vi "Joystick_test.vi"() -> ()   [LabVIEW 2017]
uses:
  NationalInstruments.VeriStand.SystemStorage
  NationalInstruments.VeriStand.SystemStorageUI
  <vilib>/Utility/file.llb/Read Delimited Spreadsheet (string).vi
  <vilib>/Utility/inputDevices.llb/joystickAcquire.vi
  <vilib>/NI Veristand/Execution/Workspace/NI VeriStand - Set Multiple Channel Values.vi
  <vilib>/NI Veristand/Execution/Workspace/NI_VS Workspace ExecutionAPI.lvlib
  <vilib>/NI Veristand/UI Controls/Single Node Browser/NI_VS UI Single Node Browser.lvlib
panel:
  in  "Single Node Browser":refnum<k24>
  out "FChannel":string[](array[string])
  out "Joystick Values":i32[](array[numeric])
  out "error out":errorcluster
  in  "Random?":bool=TRUE
  in  "Stop":bool
  in  "NIVS.System Definition Root":refnum<k24>
  in  "NIVS.Project File Path":path
  in  "NIVS.Workspace Event":refnum<event-registration>
  in  "NIVS.Gateway IP Address":string
  in  "NIVS.INI File Path":path
  # "Use this example as a template to create custom tools for the NI VeriStand Workspace. This example shows the use of the NI VeriStand API and UI controls to set and get data.\n\nRun this example by adding this VI as a Workspace Tool item. For Help adding Workspace Tool items, please reference the NI VeriStand Help."
  # "This is the file path to the VeriStand system definition file. You can read or write to the file using the System Definition API."
  # "This is the root reference to the active System Definition file. You could use this to read the configuration or populate a tree with channels. You are free to close this reference, but it will be closed for you if you don't."
  # "This is the IP Address of the VeriStand Gateway to which the Workspace is connected. Use this to open all the .NET Manager references. Usually the Gateway is running on localhost, but it could be running on a neighbor's machine."
  # "This registered string User Event is used to help instruct your tool to shut down when the Workspace is closing."
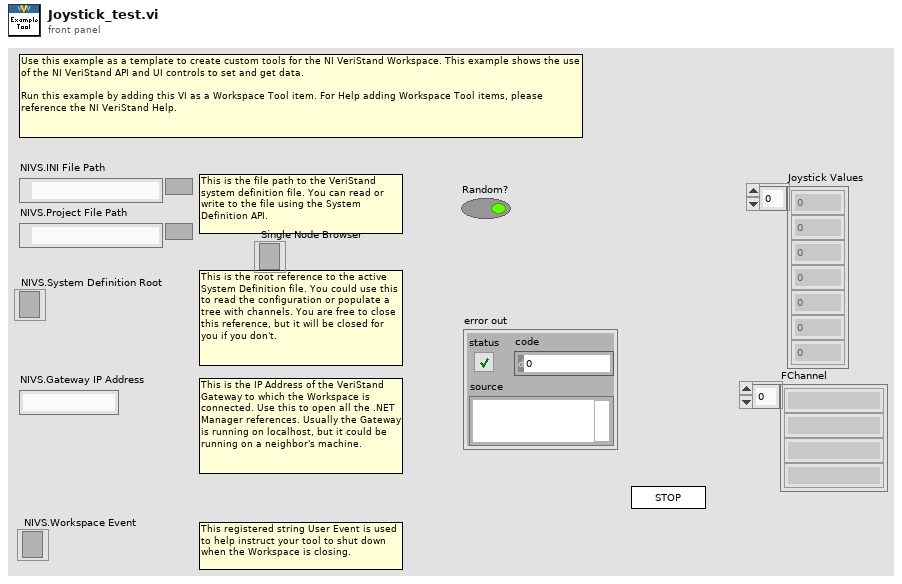
[diagram p1: front panel]
types:
  T1 = typedef "NI_VS UI Single Node Browser.lvlib/Callback Type.ctl" = cluster{"Net Callbacks":refnum<k27>[], "Event":refnum<user-event>}
  T2 = typedef "NI_VS Workspace ExecutionAPI.lvlib/WorkspaceAPI.ctl" = refnum<k24>
  T3 = typedef "NI_VS Workspace ExecutionAPI.lvlib/SystemStateEventRef.ctl" = cluster{"CustDatRef":refnum<user-event>, "EvtRef":refnum<k27>, "Target State User Event":refnum<user-event>}
  T4 = typedef "NI_VS Workspace ExecutionAPI.lvlib/SystemStateRegEventRef.ctl" = refnum<event-registration>
  T5 = cluster{"NIVS.Workspace Event":refnum<event-registration>, "Event Registration Refnum":refnum<event-registration>, "SystemChangeEventRef":T4}
  T6 = cluster{"X axis":i32, "Y axis":i32, "Z axis":i32, "X axis rotation":i32, "Y axis rotation":i32, "Z axis rotation":i32, "U axis":i32, "V axis":i32}
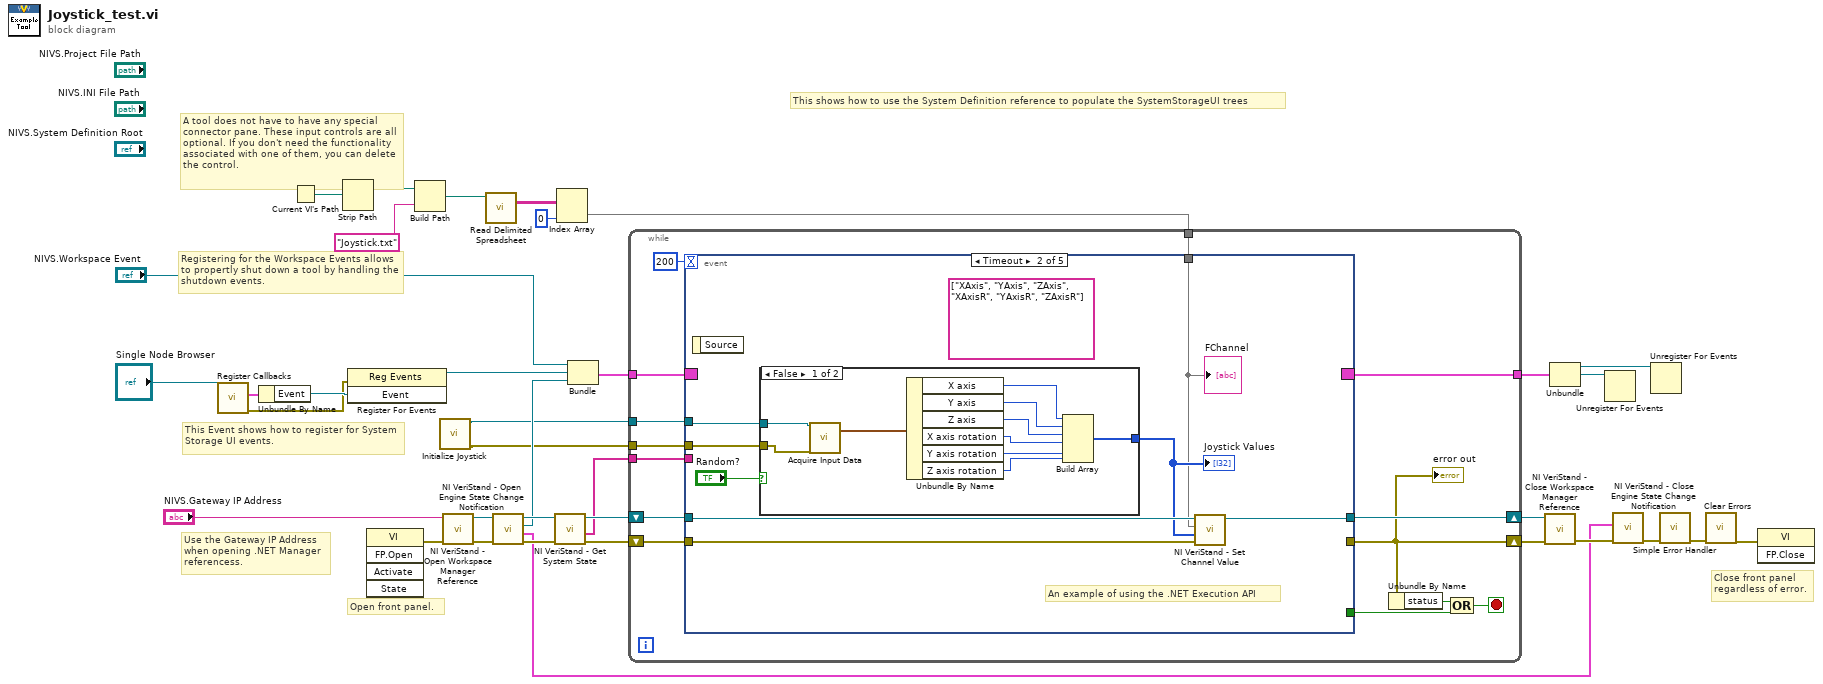
[diagram p0: block diagram]
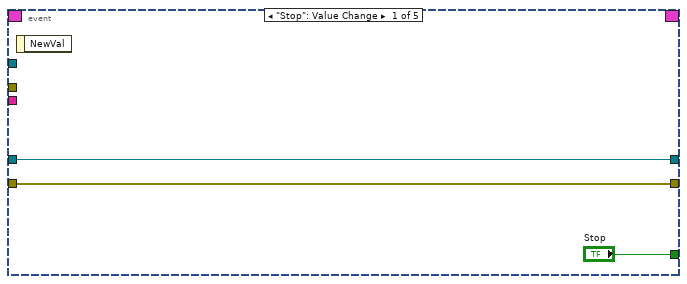
[diagram p2: hidden frame]
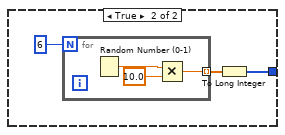
[diagram p3: hidden frame]
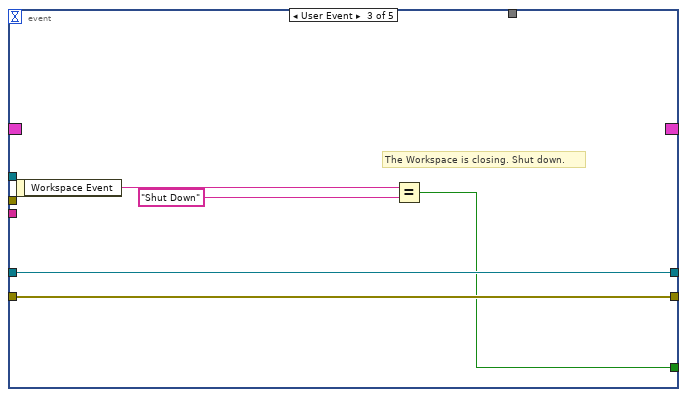
[diagram p4: hidden frame]
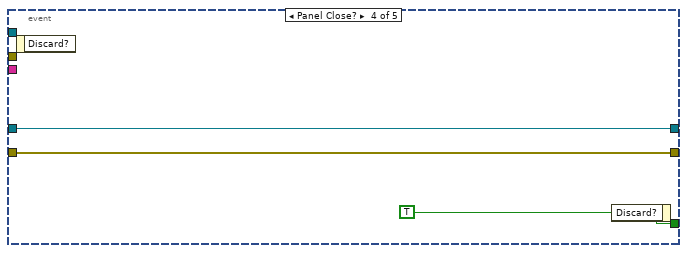
[diagram p5: hidden frame]
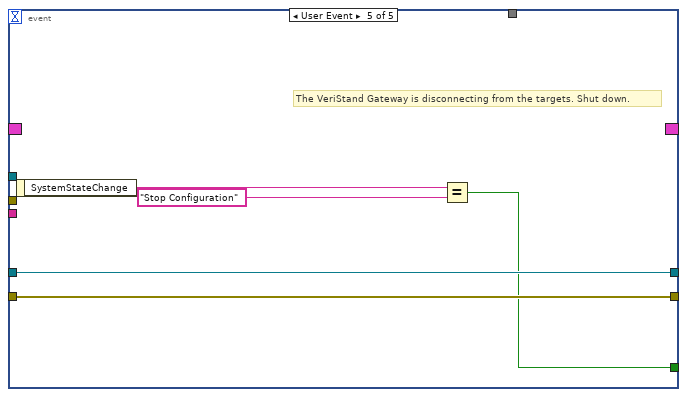
[diagram p6: hidden frame]
diagram:
  # "This Event shows how to register for System Storage UI events."
  # "Use the Gateway IP Address when opening .NET Manager referencess."
  # "A tool does not have to have any special connector pane. These input controls are all optional. If you don't need the functionality associated with one of them, you can delete the control."
  # "This shows how to use the System Definition reference to populate the SystemStorageUI trees"
  # "Registering for the Workspace Events allows to propertly shut down a tool by handling the shutdown events."
  # "Close front panel\nregardless of error."
  # "Open front panel."
  n1 = call <vilib>:"Register Callbacks.vi"("Single Node Browser"="Single Node Browser") -> ("error out"=w1:errorcluster, "Callbacks"=w12:T1)  [unwired: 8 in, 1 out]
  n2 = Unbundle By Name(w12) -> ("Event"=w11:refnum<user-event>)
  n3 = Current VI's Path() -> (path=w10:path)
  n4 = Strip Path(path=w10) -> (stripped path=w9:path)  [unwired: 1 out]
  n5 = register-events(error in=w1, w11) -> (reference out=w15:refnum<event-registration>)  [unwired: 1 in, 1 out]
  n6 = invoke class="VI" method="FP.Open"() -> (error out=w19:errorcluster)  [unwired: 5 in, 4 out]
  n7 = Build Path(base path=w9, name or relative path="Joystick.txt") -> (appended path=w7:path)
  n8 = call <vilib>:"Initialize Joystick.vi"() -> ("error out"=w2:errorcluster, "device ID"=w3:refnum<k1>)  [unwired: 10 in]
  n9 = call <vilib>:"NI VeriStand - Open Workspace Manager Reference.vi"("error in (no error)"=w19, "Gateway IP Address (\"\": localhost)"="NIVS.Gateway IP Address") -> ("error out"=w30:errorcluster, "WorkspaceManager"=w31:T2)  [unwired: 8 in]
  n10 = call-poly <vilib>:"Read Delimited Spreadsheet.vi"("file path (dialog if empty)"=w7) -> ("all rows"=w6:string[][])  [unwired: 9 in, 5 out]
  n11 = call <vilib>:"NI VeriStand - Open Engine State Change Notification.vi"("error in (no error)"=w30, "WorkspaceManager in"=w31) -> ("error out"=w35:errorcluster, "SystemStateRefs"=w24:T3, "SystemChangeEventRef"=w14:T4, "WorkspaceManager out"=w36:T2)  [unwired: 6 in]
  n12 = call <vilib>:"NI VeriStand - Get System State.vi"("error in (no error)"=w35, "WorkspaceManager in"=w36) -> ("error out"=w22:errorcluster, "Targets"=w21:string[], "WorkspaceManager  out"=w23:T2)  [unwired: 5 in, 2 out]
  n13 = Index Array(array=w6, index (col)=0 ("disabled index (col)")) -> (element=w4:string[])  [unwired: 1 in]
  n14 = Bundle("NIVS.Workspace Event"="NIVS.Workspace Event", "Event Registration Refnum"=w15, "SystemChangeEventRef"=w14) -> (w29:T5)  [unwired: 1 in]
  n15 = while {
    tunnel: w29 -> [w50]
    tunnel: [w49] -> w28
    shift-right: [w42] -> w32
    shift-left: w22 -> [w47]
    shift-right: [w46] -> w33
    shift-left: w23 -> [w48]
    tunnel: w21 -> [w44]
    tunnel: w2 -> [w39]
    tunnel: w3 -> [w38]
    tunnel: w4 -> [w37]
    stop <- w40 stop-if-true
    n16 = event shown="[1] Timeout" {
      selector: w50 -> [_ _ _ _ _]
      dyn-events: [_ _ _ _ _] -> w49
      timeout: 200 -> [_ _ _ _ _]
      tunnel: ["Stop" _ w78 w83 w86] -> w41
      tunnel: w48 -> [w52 w61 w81 w84 w89]
      tunnel: w47 -> [w53 w60 w82 w85 w90]
      tunnel: [w53 _ w82 w85 w90] -> w42
      tunnel: [w52 w59 w81 w84 w89] -> w46
      tunnel: w44 -> [_ _ _ _ _]
      tunnel: w39 -> [_ w56 _ _ _]
      tunnel: w38 -> [_ w58 _ _ _]
      tunnel: w37 -> [_ w54 _ _ _]
      event "Stop": Value Change {
        n17 = event-data() -> ()  [unwired: 1 in, 1 out]
      }
      event Timeout {
        (unwired) string[] ["XAxis", "YAxis", "ZAxis", "XAxisR", "YAxisR", "ZAxisR"] ("Channels")
        # "An example of using the .NET Execution API"
        n18 = event-data() -> ()  [unwired: 1 in, 1 out]
        n19 = case shown="False" "Random?" {
          tunnel: [w65 w72] -> w57
          tunnel: w58 -> [w64 _]
          tunnel: w56 -> [w63 _]
          frame False {
            n20 = call-poly <vilib>:"Acquire Input Data.vi"("device ID"=w64, "error in (no error)"=w63) -> ("axis info"=w62:T6)  [unwired: 13 in, 4 out]
            n21 = Unbundle By Name(w62) -> ("X axis"=w71:i32, "Y axis"=w70:i32, "Z axis"=w69:i32, "X axis rotation"=w68:i32, "Y axis rotation"=w67:i32, "Z axis rotation"=w66:i32)
            n22 = Build Array(w71, w70, w69, w68, w67, w66) -> (w65:i32[])
          }
          frame True {
            n23 = for {
              N: 6 -> [_]
              tunnel: [w76] -> w74 mode=indexing
              n24 = Random Number (0-1)() -> (number: 0 to 1=w77:dbl)
              n25 = Multiply(x=w77, y=10.0) -> (x*y=w76:dbl)
            }
            n26 = To Long Integer(number=w74) -> (32bit integer=w72:i32[])
          }
        }
        "Joystick Values" <- w57
        n27 = call-poly <vilib>:"NI VeriStand - Set Channel Value.vi"("error in (no error)"=w60, "Values"=w57, "Channels"=w54, "WorkspaceManager in"=w61) -> ("WorkspaceManager out"=w59:T2)  [unwired: 6 in, 1 out]
        "FChannel" <- w54
      }
      event User Event {
        # "The Workspace is closing. Shut down."
        n28 = event-data() -> ("Workspace Event"=w80:string)  [unwired: 1 in]
        n29 = Equal?(x=w80, y="Shut Down") -> (x = y?=w78:bool)
      }
      event Panel Close? {
        w83 = TRUE ("Discard?")
        n30 = event-data() -> ()  [unwired: 1 in, 1 out]
        n31 = event-data("Discard?"=w83) -> ()  [unwired: 1 in, 1 out]
      }
      event User Event {
        # "The VeriStand Gateway is disconnecting from the targets. Shut down."
        n32 = event-data() -> ("SystemStateChange"=w88:string)  [unwired: 1 in]
        n33 = Equal?(x=w88, y="Stop Configuration") -> (x = y?=w86:bool)
      }
    }
    "error out" <- w42
    n34 = Unbundle By Name(w42) -> ("status"=w43:bool)
    n35 = Compound Arithmetic op=OR(w43, w41) -> (w40:bool)
  }
  n36 = call <vilib>:"NI VeriStand - Close Workspace Manager Reference.vi"("error in (no error)"=w32, "WorkspaceManager"=w33) -> ("error out"=w25:errorcluster)  [unwired: 9 in]
  n37 = Unbundle(w28) -> ("NIVS.Workspace Event"=w26:refnum<event-registration>, "Event Registration Refnum"=w27:refnum<event-registration>)  [unwired: 1 out]
  n38 = Unregister For Events(event registration refnum=w27) -> ()  [unwired: 1 in, 1 out]
  n39 = call <vilib>:"NI VeriStand - Close Engine State Change Notification.vi"("error in (no error)"=w25, "SystemStateRefs"=w24) -> ("error out"=w18:errorcluster)  [unwired: 9 in]
  n40 = Unregister For Events(event registration refnum=w26) -> ()  [unwired: 1 in, 1 out]
  n41 = call <vilib>:"Simple Error Handler.vi"("error in (no error)"=w18) -> ("error out"=w17:errorcluster)  [unwired: 4 in, 4 out]
  n42 = call <vilib>:"Clear Errors.vi"("error in (no error)"=w17) -> ("error out"=w16:errorcluster)  [unwired: 5 in, 1 out]
  n43 = invoke class="VI" method="FP.Close"(error in=w16) -> ()  [unwired: 2 in, 3 out]
